vi "test.from.str.Time.vi"() -> ()   [LabVIEW 2020]
uses:
  fpga/orderbook.command.ctl
  fpga/orderbook.command.type.ctl
  fpganow.common.host.lvlib
  fpga/fpganow.common.fpga.lvlib
panel:
  out "Actual out":T1 {"symbol" format="%.0x"; "orderId" format="%.0x"}
  in  "Expected out":T1={"type"=enum."Time", "side"=0, "orderId "=13758425324623625965, "quantity"=0, "symbol"=18369548393097576175, "price"=0, "executed.qty"=0, "canceled.qty"=0, "remaining.qty"=0, "seconds"=44700, "nanoseconds"=0, "Add"=FALSE, "Edit"=FALSE, "Remove"=FALSE, "seq no"=0, "recv.time"=0, "parse.time"=0} {"symbol" format="%.0x"; "orderId" format="%.0x"}
  in  "String in":string="(Time, 44700)"
  out "Passed?":bool
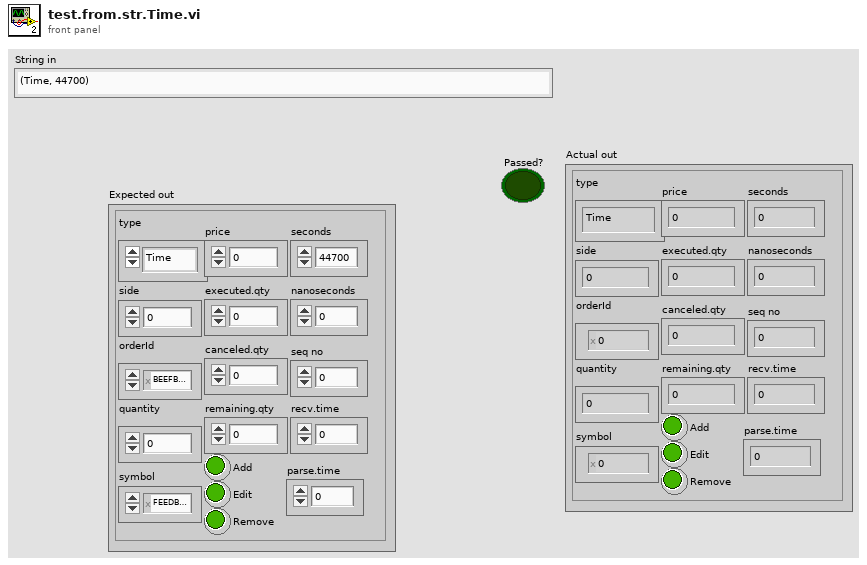
[diagram p1: front panel]
types:
  T1 = typedef "fpganow.common.fpga.lvlib/orderbook.command.ctl" = cluster{"type":T2, "side":u8, "orderId ":u64, "quantity":u32, "symbol":u64, "price":u64, "executed.qty":u32, "canceled.qty":u32, "remaining.qty":u32, "seconds":u64, "nanoseconds":u64, "Add":bool, "Edit":bool, "Remove":bool, "seq no":u32, "recv.time":u64, "parse.time":u64}
  T2 = typedef "fpganow.common.fpga.lvlib/orderbook.command.type.ctl" = enum8{"Time", "AddOrder", "OrderExecuted", "OrderExecutedAtPrice", "ReduceSize", "ModifyOrder", "DeleteOrder", "Get.Everything", "Get.All.Orders", "Get.Top"}
  T3 = cluster{"type":bool, "side":bool, "orderId ":bool, "quantity":bool, "symbol":bool, "price":bool, "executed.qty":bool, "canceled.qty":bool, "remaining.qty":bool, "seconds":bool, "nanoseconds":bool, "Add":bool, "Edit":bool, "Remove":bool, "seq no":bool, "recv.time":bool, "parse.time":bool}
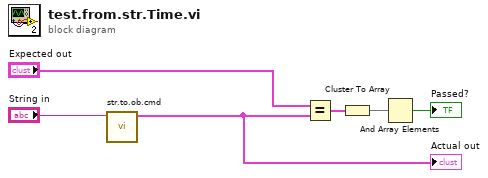
[diagram p0: block diagram]
diagram:
  n1 = call "str.to.ob.cmd.vi"("string in"="String in") -> ("orderbook.command"=w4:T1)  [unwired: 10 in]
  "Actual out" <- w4
  n2 = Equal?(x="Expected out", y=w4) -> (x = y?=w3:T3)
  n3 = Cluster To Array(cluster=w3) -> (array=w2:bool[])
  n4 = And Array Elements(Boolean array=w2) -> (logical AND=→"Passed?":bool)
